vi "Apply_Power_Control_Setpoints_16.vi"(0 "SI804.lvclass":refnum<class "SI804.lvclass">, 2 "3 JSD20 FG412\nXA01":bool, 3 "3 JSD40 FX110\nXA01":bool, 4 "3 JSB30 FD711\nXA01":bool, 5 "error in":errorcluster) -> (14 "SI804.lvclass out":refnum<class "SI804.lvclass">, 16 "Apply L-Bank SP":bool, 17 "Apply PD SP":bool, 18 "Apply Boron SP":bool, 19 "error out":errorcluster)   [LabVIEW 2022 SP3, in "SI804.lvclass"]
uses:
  SI804.lvclass
  SI804.lvclass/SI804.ctl
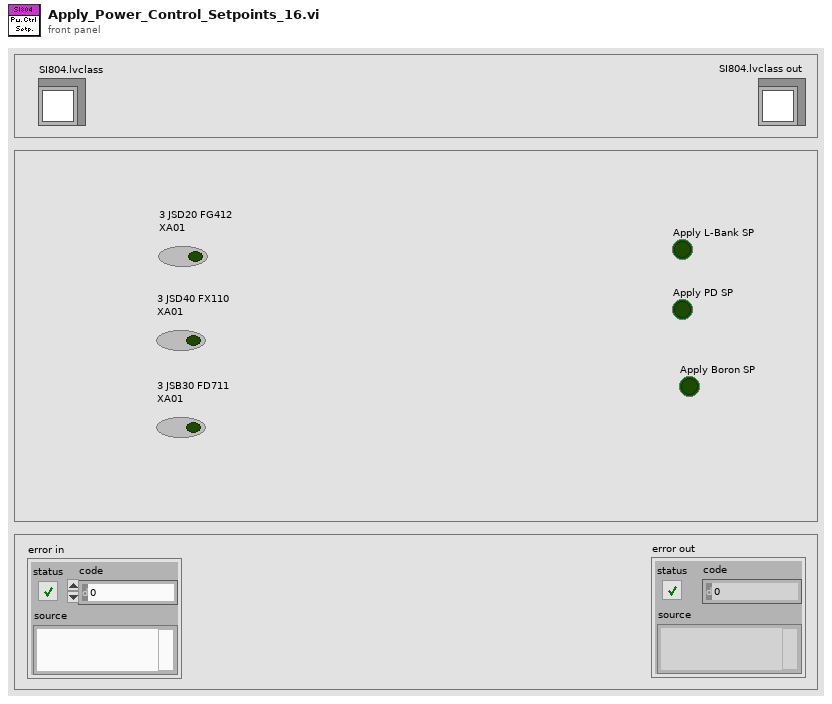
[diagram p1: front panel]
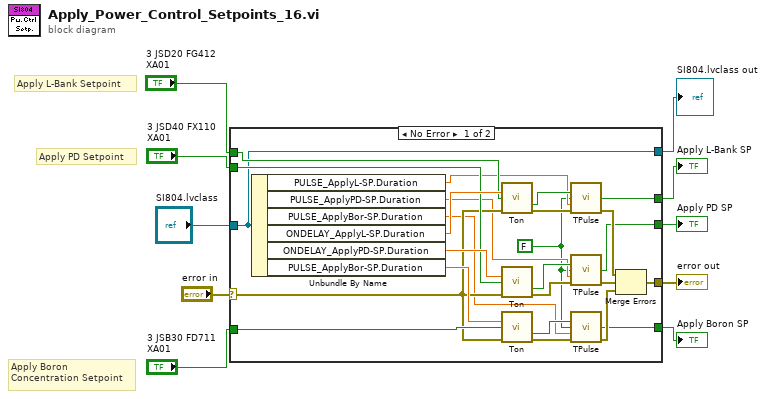
[diagram p0: block diagram]
diagram:
  # "Apply Boron\nConcentration Setpoint"
  # "Apply PD Setpoint"
  # "Apply L-Bank Setpoint"
  n1 = case shown="No Error" "error in" {
    selector: "error in" -> [w29 w36]
    tunnel: "3 JSD20 FG412\nXA01" -> [w32 _]
    tunnel: "3 JSD40 FX110\nXA01" -> [w31 _]
    tunnel: "3 JSB30 FD711\nXA01" -> [w30 _]
    tunnel: "SI804.lvclass" -> [w11 w37]
    tunnel: [w19 w36] -> w5
    tunnel: [w18 _] -> w3
    tunnel: [w17 _] -> w2
    tunnel: [w16 _] -> w1
    tunnel: [w11 w37] -> w4
    frame No Error {
      w12 = FALSE ("Reset")
      n2 = Unbundle By Name(w11) -> ("PULSE_ApplyL-SP.Duration"=w15:dbl, "PULSE_ApplyPD-SP.Duration"=w14:dbl, "PULSE_ApplyBor-SP.Duration"=w13:dbl, "ONDELAY_ApplyL-SP.Duration"=w35:dbl, "ONDELAY_ApplyPD-SP.Duration"=w34:dbl, "PULSE_ApplyBor-SP.Duration"=w33:dbl)
      n3 = call "Ton.vi"("Ton"=w35, "input"=w32, "error in"=w29) -> ("Binary out"=w25:bool, "error out"=w28:errorcluster)  [unwired: 8 in, 3 out]
      n4 = call "Ton.vi"("Ton"=w34, "input"=w31, "error in"=w29) -> ("Binary out"=w24:bool, "error out"=w27:errorcluster)  [unwired: 8 in, 3 out]
      n5 = call "Ton.vi"("Ton"=w33, "input"=w30, "error in"=w29) -> ("Binary out"=w23:bool, "error out"=w26:errorcluster)  [unwired: 8 in, 3 out]
      n6 = call "TPulse.vi"("trigger"=w25, "Reset"=w12, "TPulse"=w15, "error in"=w28) -> ("output"=w18:bool, "error out"=w22:errorcluster)  [unwired: 9 in, 1 out]
      n7 = call "TPulse.vi"("trigger"=w24, "Reset"=w12, "TPulse"=w14, "error in"=w27) -> ("output"=w17:bool, "error out"=w21:errorcluster)  [unwired: 9 in, 1 out]
      n8 = call "TPulse.vi"("trigger"=w23, "Reset"=w12, "TPulse"=w13, "error in"=w26) -> ("output"=w16:bool, "error out"=w20:errorcluster)  [unwired: 9 in, 1 out]
      n9 = Merge Errors(w22, w21, w20) -> (w19:errorcluster)
    }
    frame Error {
    }
  }
  "error out" <- w5
  "SI804.lvclass out" <- w4
  "Apply L-Bank SP" <- w3
  "Apply PD SP" <- w2
  "Apply Boron SP" <- w1
